vi "Wrt_St_Time.vi"(8 "Error In":errorcluster, 11 "StartTimePath":path) -> (0 "Error Out":errorcluster)   [LabVIEW 2020, in "Main.lvlib"]
uses:
  Main.lvlib
  Time/Time.lvlib
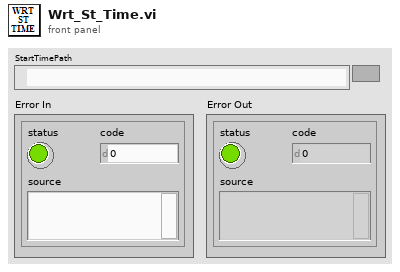
[diagram p1: front panel]
types:
  T1 = typedef "Time.lvlib/Local_DateTime_String.ctl" = cluster{"Local Date Time":string, "Local Date":string, "Local Time":string}
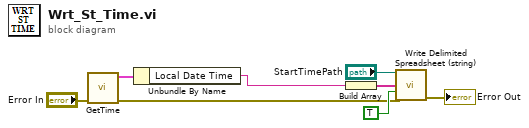
[diagram p0: block diagram]
diagram:
  n1 = call "GetTime.vi"("error in"="Error In") -> ("error out"=w3:errorcluster, "Local Data/Time[String]"=w2:T1)  [unwired: 8 in, 1 out]
  n2 = Unbundle By Name(w2) -> ("Local Date Time"=w1:string)
  n3 = Build Array(w1) -> (w8:string[])
  n4 = call "Write Delimited Spreadsheet (string).vi"("file path (dialog if empty)"="StartTimePath", "1D data"=w8, "append to file? (new file:F)"=TRUE, "error in (no error)"=w3) -> ("error out"=→"Error Out":errorcluster)  [unwired: 10 in, 1 out]
